vi "Set Position.vi"(8 "error in (no error)":errorcluster, 10 "Position":i32, 11 "FW102C in":i32) -> (0 "error out":errorcluster, 3 "FW102C out":i32)   [LabVIEW 2018, in "Thorlabs_FW102C.lvlib"]
doc: "Moves the wheel to filter position n (1-6, or 1-12)"
uses:
  Thorlabs_FW102C.lvlib
  <instrlib>/Thorlabs_FW102C/Library/FilterWheel102_win32.dll
  Library/FilterWheel102_win64.dll
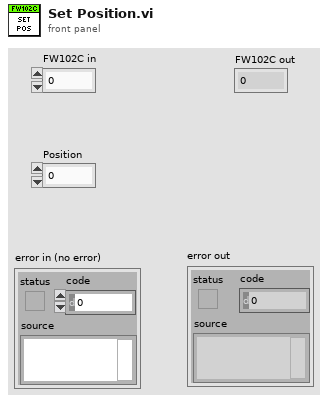
[diagram p1: front panel]
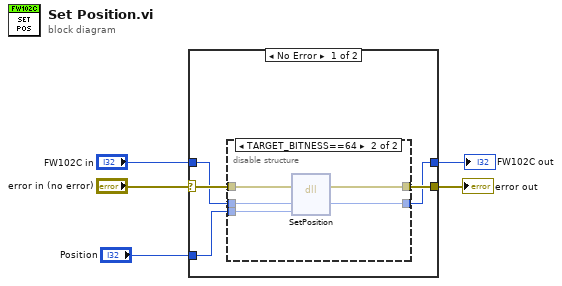
[diagram p0: block diagram]
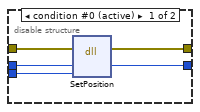
[diagram p2: hidden frame]
diagram:
  n1 = case shown="No Error" "error in (no error)" {
    selector: "error in (no error)" -> [w10 w21]
    tunnel: [w9 w21] -> w5
    tunnel: "FW102C in" -> [w8 w22]
    tunnel: [w7 w22] -> w2
    tunnel: "Position" -> [w6 _]
    frame No Error {
      n2 = disable-structure shown="TARGET_BITNESS==64" {
        disable-tunnel: w10 -> [w15 w20]
        disable-tunnel: [w14 w19] -> w9
        disable-tunnel: w8 -> [w13 w18]
        disable-tunnel: [w12 w17] -> w7
        disable-tunnel: w6 -> [w11 w16]
        frame condition #0 (active) {
          n3 = dll-call lib="E:/Program Files (x86)/National Instruments/LabVIEW 2011/instr.lib/Thorlabs_FW102C/Library/FilterWheel102_win32.dll" fn="SetPosition"(error in=w15, "hdl"=w13, "position"=w11) -> (error out=w14:errorcluster, "hdl"=w12:i32)  [unwired: 4 in, 1 out]
        }
        frame condition #1 {
          n4 = dll-call lib="C:/Users/aspitarl/Git/MHDLab/Filter Wheel/Thorlabs_FW102C/Library/FilterWheel102_win64.dll" fn="SetPosition"(error in=w20, "hdl"=w18, "position"=w16) -> (error out=w19:errorcluster, "hdl"=w17:i32)  [unwired: 4 in, 1 out]
        }
      }
    }
    frame Error {
    }
  }
  "error out" <- w5
  "FW102C out" <- w2
